vi "dataset.label_count.vi"(8 "error in":errorcluster, 11 "Dataset in":refnum<class "Dataset.lvclass">) -> (0 "error out":errorcluster, 3 "Dataset out":refnum<class "Dataset.lvclass">)   [LabVIEW 2020, in "Dataset.lvclass"]
doc: "Returns the number of labels on the dataset."
uses:
  Dataset.lvclass
  Dataset.lvclass/Dataset.ctl
  client.lvlib
panel:
  out "out_count out":u32
  in  "out_count":u32
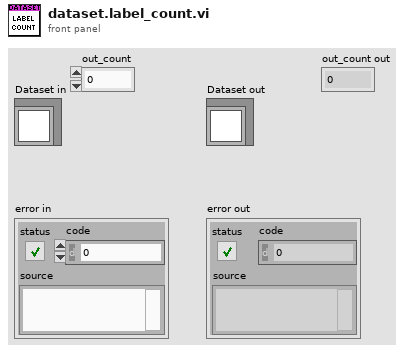
[diagram p1: front panel]
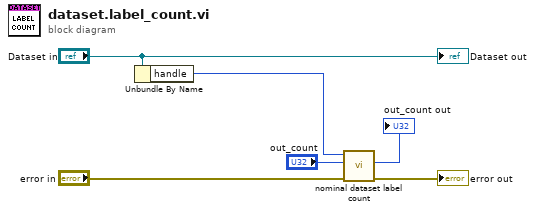
[diagram p0: block diagram]
diagram:
  n1 = Unbundle By Name("Dataset in") -> ("handle"=w4:i32)
  n2 = call "nominal dataset label count.vi"("error in (no error)"="error in", "out_count"="out_count", "dataset"=w4) -> ("error out"=→"error out":errorcluster, "out_count out"=→"out_count out":u32)  [unwired: 6 in, 1 out]
  "Dataset out" <- "Dataset in"
